vi "calculation vi_grMD.vi"() -> ()   [LabVIEW 2017]
doc: "SciScan 1.1f2 160418"
uses:
  CommonResource VIs/Timing/Timer Commands.ctl
  <vilib>/Utility/VariantDataType/Type.ctl
  GFG/GFGfpRefGet.vi
  GFG/GFG library.lvlib
  <vilib>/Utility/VariantDataType/VariantType.lvlib
panel:
  out "Source VI":string
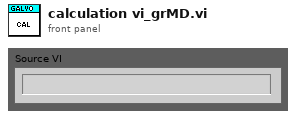
[diagram p1: front panel]
types:
  T1 = typedef "Timer Commands.ctl" = enum16{"Clear All", "Start", "Pause", "Check Time"}
  T2 = cluster{"WaveformChartRef":refnum<vi>, "DigitalRef":refnum<vi>, "ArrayRef":refnum<vi>, "TabControlRef":refnum<vi>, "EnumRef":refnum<vi>, "RingRef":refnum<vi>, "BooleanRef":refnum<vi>, "KnobRef":refnum<vi>, "SlideRef":refnum<vi>, "PathRef":refnum<vi>, "StringRef":refnum<vi>, "ComboBox":refnum<vi>, "WaveformGraphRef":refnum<vi>}
  T3 = enum8{"Enabled", "Disabled", "Disabled and Grayed Out"}
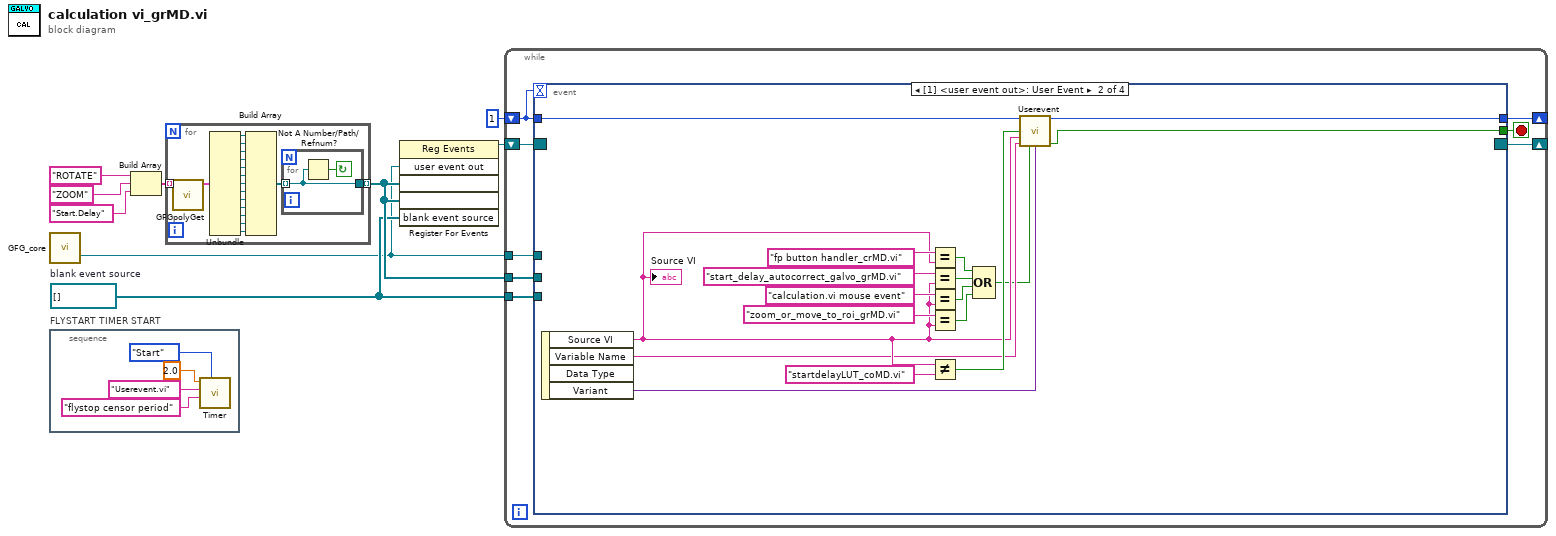
[diagram p0: block diagram]
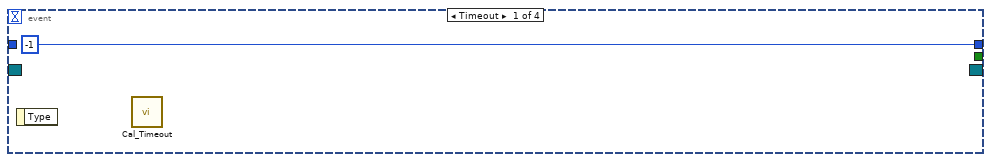
[diagram p2: hidden frame]
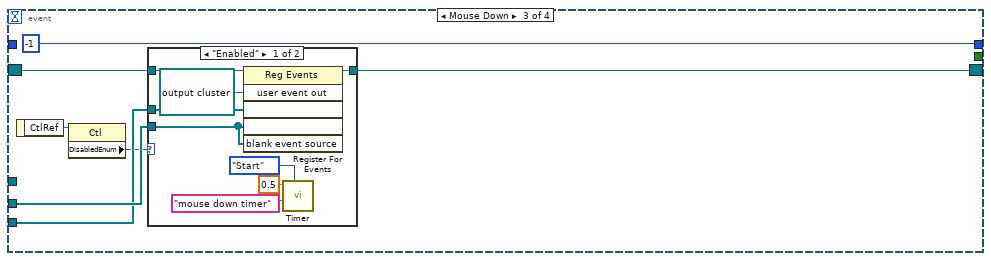
[diagram p3: hidden frame]
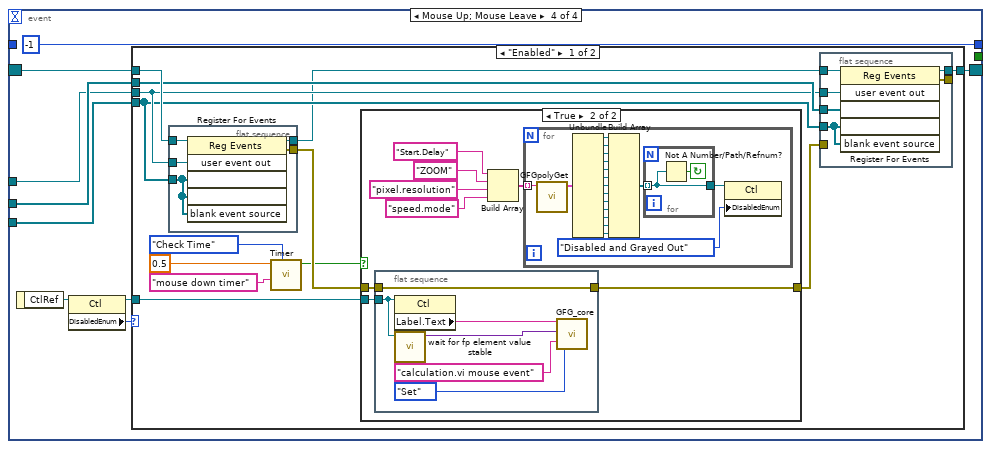
[diagram p5: hidden frame]
diagram:
  w2 = refnum<vi>[] []  # blank event source
  n1 = call "GFG_core.vi"() -> ("user event out"=w1:refnum<user-event>)  [unwired: 13 in, 6 out]
  n2 = stacked-sequence "FLYSTART TIMER START" {
    frame #0 {
      n3 = call "Timer.vi"("Timer Command"=Timer_Commands."Start", "name qualifier (empty if unwired)"="flystop censor period", "VI name (Optional)"="Userevent.vi" ("name qualifier (empty if unwired)"), "Set Time IN (s)"=2.0) -> ()  [unwired: 2 in, 6 out]
    }
  }
  n4 = Build Array("ROTATE", "ZOOM", "Start.Delay") -> (w8:string[])
  n5 = for {
    tunnel: w8 -> [w30] mode=indexing
    tunnel: [w14] -> w3 mode=indexing
    n6 = call-poly "GFGpolyGet.vi"("Variable Name in"=w30) -> ("output cluster"=w16:T2)  [unwired: 9 in, 1 out]
    n7 = Unbundle(w16) -> ("WaveformChartRef"=w27:refnum<vi>, "DigitalRef"=w26:refnum<vi>, "ArrayRef"=w25:refnum<vi>, "TabControlRef"=w24:refnum<vi>, "EnumRef"=w23:refnum<vi>, "RingRef"=w22:refnum<vi>, "BooleanRef"=w21:refnum<vi>, "KnobRef"=w20:refnum<vi>, "SlideRef"=w19:refnum<vi>, "PathRef"=w18:refnum<vi>, "StringRef"=w17:refnum<vi>, "ComboBox"=w28:refnum<vi>, "WaveformGraphRef"=w29:refnum<vi>)
    n8 = Build Array(w27, w26, w25, w24, w23, w22, w21, w20, w19, w18, w17, w28, w29) -> (w15:refnum<vi>[])
    n9 = for {
      tunnel: w15 -> [w31] mode=indexing
      tunnel: [w31] -> w14
      stop <- w32 continue-if-true
      n10 = Not A Number/Path/Refnum?(number/path/refnum=w31) -> (NaN/Path/Refnum?=w32:bool)
    }
  }
  n11 = register-events(w1, w3, w3, w2) -> (reference out=w4:refnum<event-registration>)  [unwired: 2 in, 1 out]
  n12 = while {
    shift-right: [w40] -> _
    shift-left: 1 -> [w39]
    tunnel: w3 -> [w38]
    shift-right: [w37] -> _
    shift-left: w4 -> [w36]
    tunnel: w1 -> [w35]
    tunnel: w2 -> [w34]
    stop <- w33 stop-if-true
    n13 = event shown="[1] <user event out>: User Event" {
      selector: w36 -> [_ _ w65 w83]
      dyn-events: [_ _ w63 w79] -> w37
      timeout: w39 -> [_ _ _ _]
      tunnel: [_ w42 _ _] -> w33
      tunnel: [-1 w43 -1 -1] -> w40
      tunnel: w39 -> [_ w49 _ _]
      tunnel: w38 -> [_ _ w64 w82]
      tunnel: w35 -> [_ _ _ w81]
      tunnel: w34 -> [_ _ w62 w80]
      event Timeout {
        n14 = event-data() -> ()  [unwired: 1 in, 1 out]
        n15 = call "Cal_Timeout.vi"() -> ()  [unwired: 12 in]
      }
      event User Event {
        n16 = event-data() -> ("Source VI"=w47:string, "Variable Name"=w46:string, "Variant"=w44:variant)  [unwired: 1 in, 1 out]
        "Source VI" <- w47
        n17 = Equal?(x="fp button handler_crMD.vi" ("y"), y=w47) -> (x = y?=w57:bool)
        n18 = Equal?(x="start_delay_autocorrect_galvo_grMD.vi" ("y"), y=w47) -> (x = y?=w55:bool)
        n19 = Equal?(x="calculation.vi mouse event" ("Source VI"), y=w47) -> (x = y?=w52:bool)
        n20 = Equal?(x="zoom_or_move_to_roi_grMD.vi" ("Source VI"), y=w47) -> (x = y?=w50:bool)
        n21 = Not Equal?(x=w47, y="startdelayLUT_coMD.vi") -> (x != y?=w48:bool)
        n22 = Compound Arithmetic op=OR(w57, w55, w52, w50) -> (w45:bool)
        n23 = call "Userevent.vi"("Timeout IN"=w49, "Source # startdelayLUT_coMD.vi?"=w48, "Source VI"=w47, "Variable name"=w46, "VI Match"=w45, "Value"=w44) -> ("Timeout OUT"=w43:i32, "shutdown?"=w42:bool)  [unwired: 8 in]
      }
      event Mouse Down {
        n24 = event-data() -> ("CtlRef"=w60:refnum<vi>)  [unwired: 1 in]
        n25 = property class="Ctl"(reference=w60) -> ("DisabledEnum"=w59:T3)  [unwired: 1 in, 2 out]
        n26 = case shown="\"Enabled\"" w59 {
          tunnel: w65 -> [w73 w74]
          tunnel: w64 -> [w72 _]
          tunnel: [w71 w74] -> w63
          tunnel: w62 -> [w70 _]
          frame "Enabled" {
            n27 = register-events(reference=w73, refnum<user-event> refnum ("user event out"), w70, w72, w72) -> (reference out=w71:refnum<event-registration>)  [unwired: 1 in, 1 out]
            n28 = call "Timer.vi"("Timer Command"=Timer_Commands."Start", "name qualifier (empty if unwired)"="mouse down timer", "Set Time IN (s)"=0.5) -> ()  [unwired: 3 in, 6 out]
          }
          frame "Disabled", Default {
          }
        }
      }
      event Mouse Up; Mouse Leave {
        n29 = event-data() -> ("CtlRef"=w77:refnum<vi>)  [unwired: 1 in]
        n30 = property class="Ctl"(reference=w77) -> (reference out=w75:refnum<vi>, "DisabledEnum"=w76:T3)  [unwired: 1 in, 1 out]
        n31 = case shown="\"Enabled\"" w76 {
          tunnel: w83 -> [w96 w143]
          tunnel: w82 -> [w95 _]
          tunnel: w81 -> [w94 _]
          tunnel: w80 -> [w93 _]
          tunnel: [w92 w143] -> w79
          tunnel: w75 -> [w84 _]
          frame "Enabled" {
            n32 = flat-sequence {
              tunnel: w96 -> [w142]
              tunnel: [w141] -> w91
              tunnel: w94 -> [w140]
              tunnel: w93 -> [w138]
              tunnel: [w139] -> w90
              frame #0 {
                n33 = register-events(reference=w142, w140, w138, w138, w138) -> (reference out=w141:refnum<event-registration>, error out=w139:errorcluster)  [unwired: 1 in]
              }
            }
            n34 = call "Timer.vi"("Timer Command"=Timer_Commands."Check Time", "name qualifier (empty if unwired)"="mouse down timer", "Set Time IN (s)"=0.5) -> ("Complete?"=w85:bool)  [unwired: 3 in, 5 out]
            n35 = case shown="True" w85 {
              tunnel: w84 -> [_ w105]
              tunnel: w90 -> [w97 w104]
              tunnel: [w97 w103] -> w89
              frame False {
              }
              frame True {
                n36 = flat-sequence {
                  tunnel: w105 -> [w131]
                  tunnel: [w126] -> w103
                  tunnel: w104 -> [w126]
                  frame #0 {
                    n37 = property class="Ctl"(reference=w131) -> ("Label.Text"=w130:string)  [unwired: 1 in, 2 out]
                    n38 = call "wait for fp element value stable.vi"("CtlRef"=w131) -> ("Value"=w129:variant)  [unwired: 9 in, 1 out]
                    n39 = call "GFG_core.vi"("Variable Name in"=w130, "Variant in"=w129, "Source VI"="calculation.vi mouse event", "Action"=enum16{"Init", "Set", "Get", "Clear"}."Set") -> ()  [unwired: 9 in, 7 out]
                  }
                }
                n40 = Build Array("Start.Delay" ("Variable Name in"), "ZOOM" ("Variable Name in"), "pixel.resolution" ("element"), "speed.mode" ("element")) -> (w98:string[])
                n41 = for {
                  tunnel: w98 -> [w123] mode=indexing
                  n42 = call-poly "GFGpolyGet.vi"("Variable Name in"=w123) -> ("output cluster"=w108:T2)  [unwired: 9 in, 1 out]
                  n43 = Unbundle(w108) -> ("WaveformChartRef"=w112:refnum<vi>, "DigitalRef"=w113:refnum<vi>, "ArrayRef"=w114:refnum<vi>, "TabControlRef"=w115:refnum<vi>, "EnumRef"=w116:refnum<vi>, "RingRef"=w117:refnum<vi>, "BooleanRef"=w118:refnum<vi>, "KnobRef"=w119:refnum<vi>, "SlideRef"=w120:refnum<vi>, "PathRef"=w121:refnum<vi>, "StringRef"=w122:refnum<vi>, "ComboBox"=w111:refnum<vi>, "WaveformGraphRef"=w110:refnum<vi>)
                  n44 = Build Array(w112, w113, w114, w115, w116, w117, w118, w119, w120, w121, w122, w111, w110) -> (w109:refnum<vi>[])
                  n45 = for {
                    tunnel: w109 -> [w124] mode=indexing
                    tunnel: [w124] -> w106
                    stop <- w125 continue-if-true
                    n46 = Not A Number/Path/Refnum?(number/path/refnum=w124) -> (NaN/Path/Refnum?=w125:bool)
                  }
                  n47 = property class="Ctl"(reference=w106, "DisabledEnum"=T3."Disabled and Grayed Out" ("Disabled")) -> ()  [unwired: 1 in, 2 out]
                }
              }
            }
            n48 = flat-sequence {
              tunnel: w91 -> [w137]
              tunnel: [w136] -> w92
              tunnel: w94 -> [w135]
              tunnel: w93 -> [w133]
              tunnel: [w134] -> _
              tunnel: w95 -> [w132]
              tunnel: w89 -> [_]
              frame #0 {
                n49 = register-events(reference=w137, w135, w132, w133, w133) -> (reference out=w136:refnum<event-registration>, error out=w134:errorcluster)  [unwired: 1 in]
              }
            }
          }
          frame "Disabled", Default {
          }
        }
      }
    }
  }
